vi "Step_Forward.vi"(3 "error in":errorcluster, 4 "Data in":T1, 5 "Step control reference in":refnum<vi>) -> (0 "error out":errorcluster, 1 "Data out":T1, 2 "Step control reference out":refnum<vi>)   [LabVIEW 2017]
uses:
  Type_Defs/Data.ctl
  Type_Defs/Diagnostics.ctl
  Type_Defs/Systems.ctl
  Step_Vis/Steps.lvlib
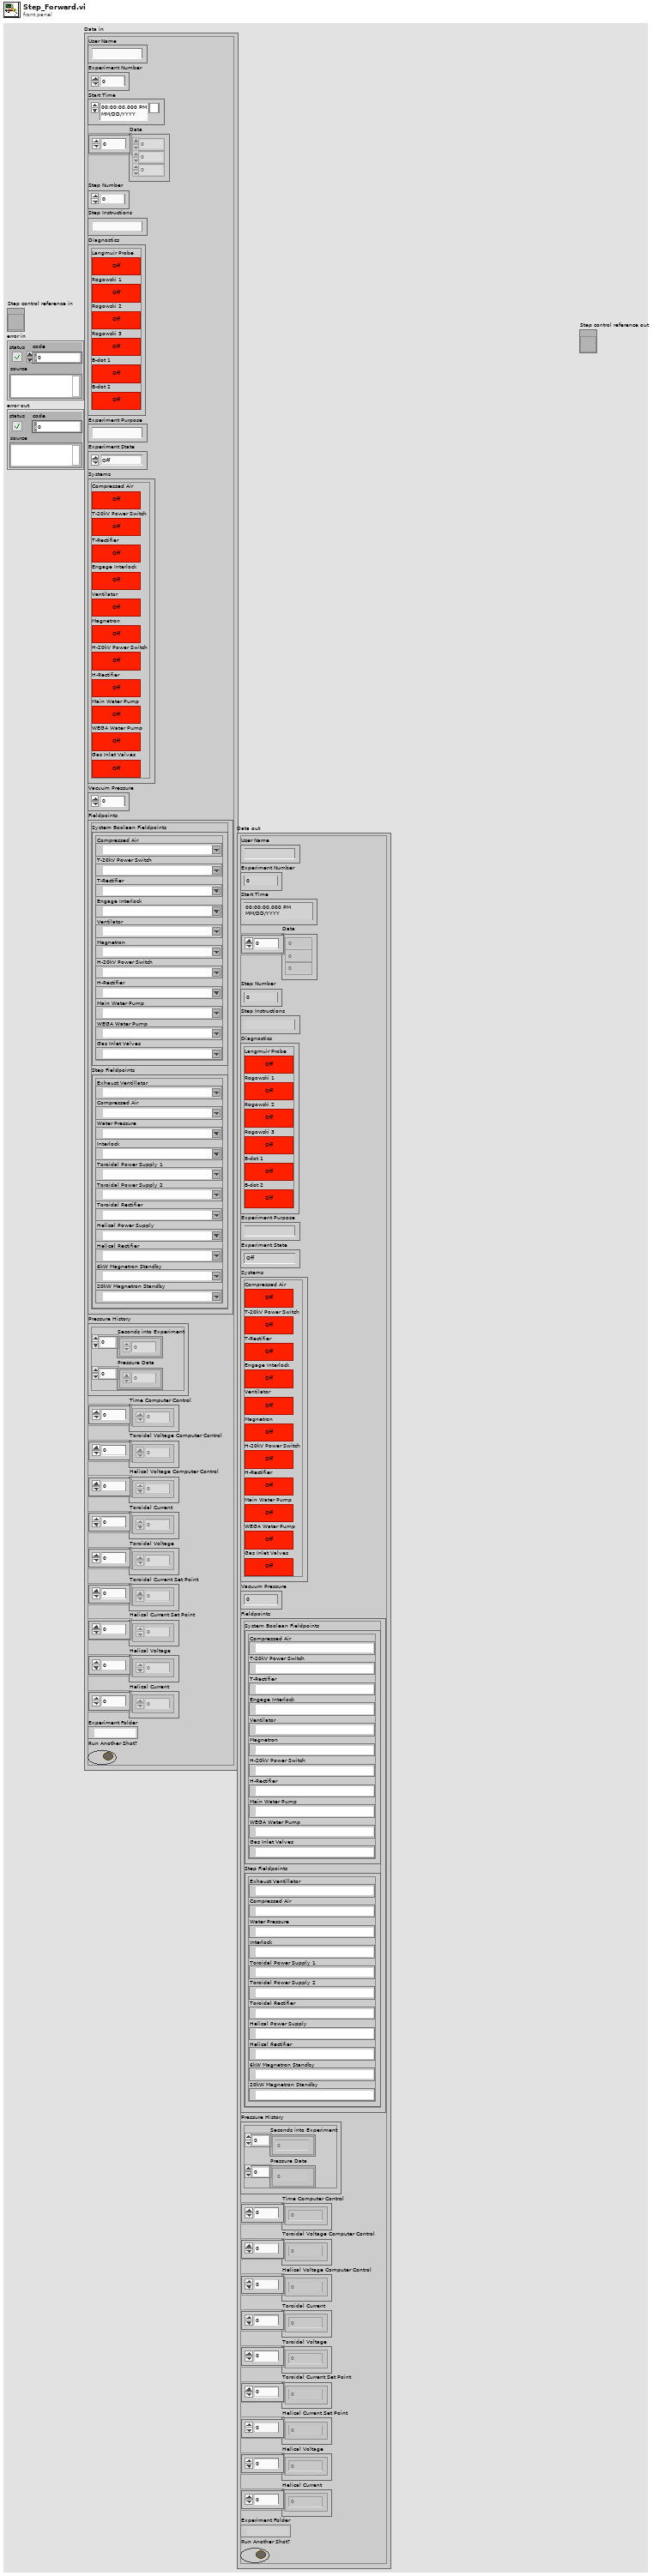
[diagram p1: front panel]
types:
  T1 = typedef "Data.ctl" = cluster{"User Name":string, "Experiment Number":i32, "Start Time":timestamp, "Data":dbl[], "Step Number":i32, "Step Instructions":string, "Diagnostics":T2, "Experiment Purpose":string, "Experiment State":enum16{"Off", "Setting Up", "Ready", "In Progress", "Shutting Down"}, "Systems":T3, "Vacuum Pressure":dbl, "Fieldpoints":cluster{"System Boolean Fieldpoints":cluster{"Compressed Air":refnum<k21>, "T-20kV Power Switch":refnum<k21>, "T-Rectifier":refnum<k21>, "Engage Interlock":refnum<k21>, "Ventilator":refnum<k21>, "Magnetron":refnum<k21>, "H-20kV Power Switch":refnum<k21>, "H-Rectifier":refnum<k21>, "Main Water Pump":refnum<k21>, "WEGA Water Pump":refnum<k21>, "Gas Inlet Valves":refnum<k21>}, "Step Fieldpoints":cluster{"Exhaust Ventillator":refnum<k21>, "Compressed Air":refnum<k21>, "Water Pressure":refnum<k21>, "Interlock":refnum<k21>, "Toroidal Power Supply 1":refnum<k21>, "Toroidal Power Supply 2":refnum<k21>, "Toroidal Rectifier":refnum<k21>, "Helical Power Supply":refnum<k21>, "Helical Rectifier":refnum<k21>, "6kW Magnetron Standby":refnum<k21>, "20kW Magnetron Standby":refnum<k21>}}, "Pressure History":cluster{"Seconds into Experiment":i32[], "Pressure Data":dbl[]}, "Time Computer Control":dbl[], "Toroidal Voltage Computer Control":dbl[], "Helical Voltage Computer Control":dbl[], "Toroidal Current":dbl[], "Toroidal Voltage":dbl[], "Toroidal Current Set Point":dbl[], "Helical Current Set Point":dbl[], "Helical Voltage":dbl[], "Helical Current":dbl[], "Experiment Folder":path, "Run Another Shot?":bool}
  T2 = typedef "Diagnostics.ctl" = cluster{"Langmuir Probe":bool, "Rogowski 1":bool, "Rogowski 2":bool, "Rogowski 3":bool, "B-dot 1":bool, "B-dot 2":bool}
  T3 = typedef "Systems.ctl" = cluster{"Compressed Air":bool, "T-20kV Power Switch":bool, "T-Rectifier":bool, "Engage Interlock":bool, "Ventilator":bool, "Magnetron":bool, "H-20kV Power Switch":bool, "H-Rectifier":bool, "Main Water Pump":bool, "WEGA Water Pump":bool, "Gas Inlet Valves":bool}
  T4 = enum16{"Off", "Setting Up", "Ready", "In Progress", "Shutting Down"}
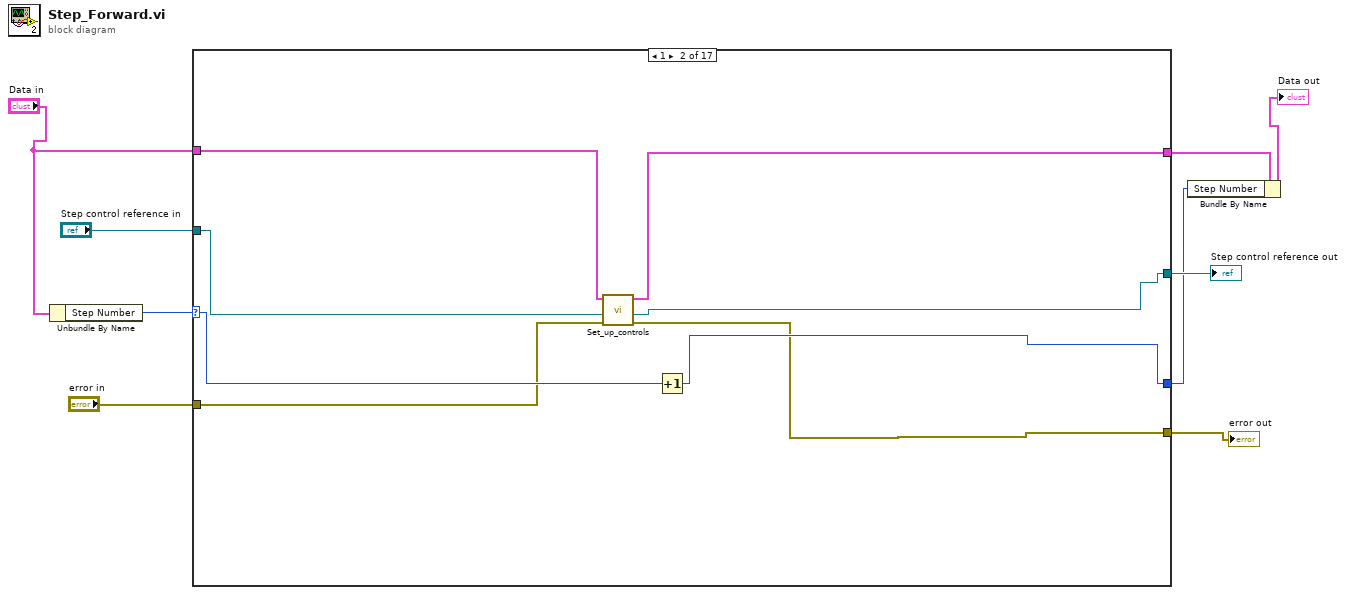
[diagram p0: block diagram]
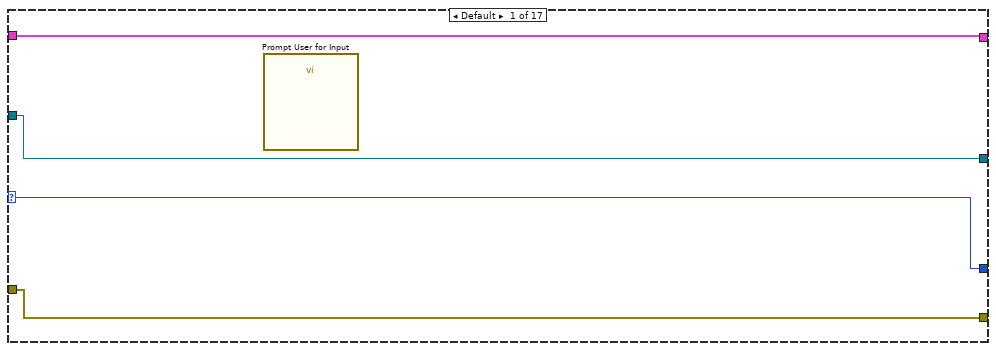
[diagram p2: hidden frame]
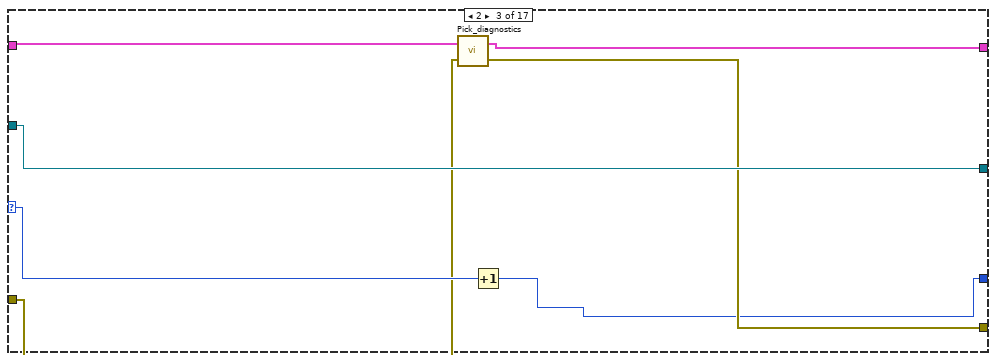
[diagram p3: hidden frame]
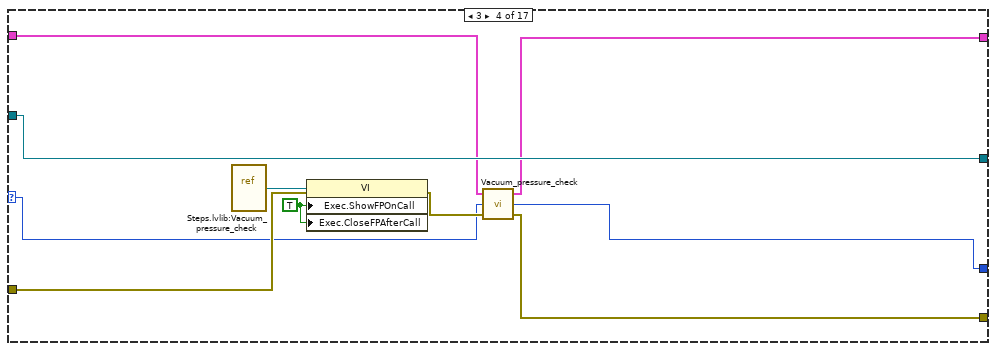
[diagram p4: hidden frame]
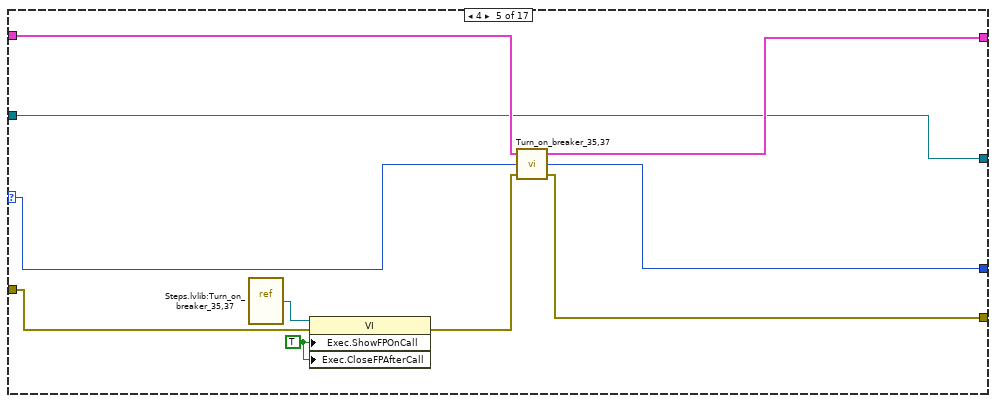
[diagram p5: hidden frame]
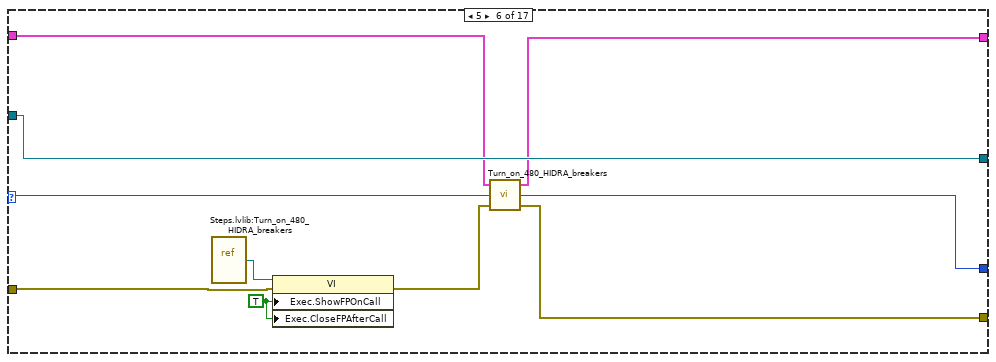
[diagram p6: hidden frame]
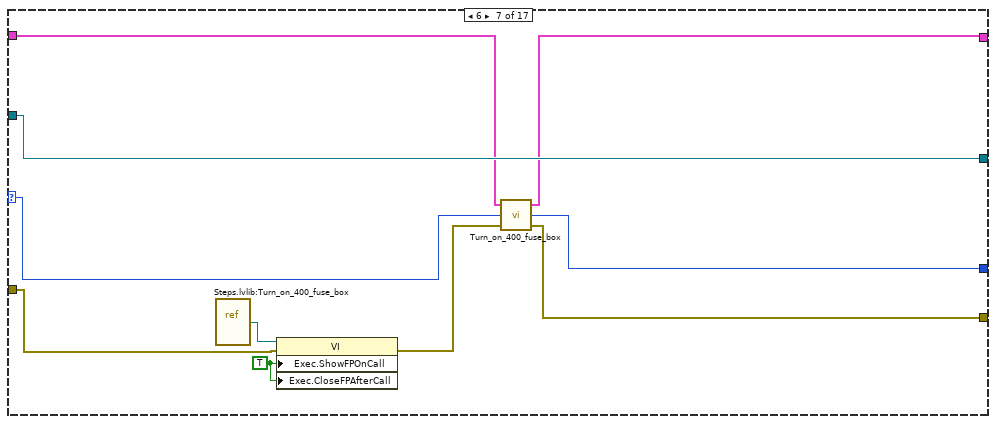
[diagram p7: hidden frame]
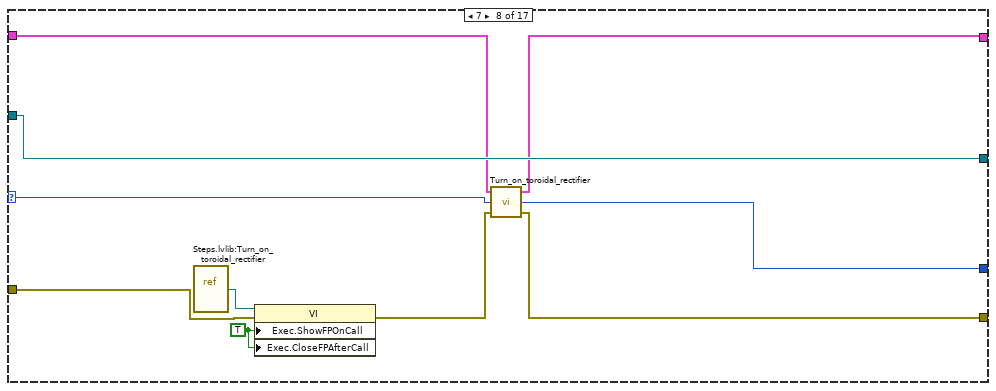
[diagram p8: hidden frame]
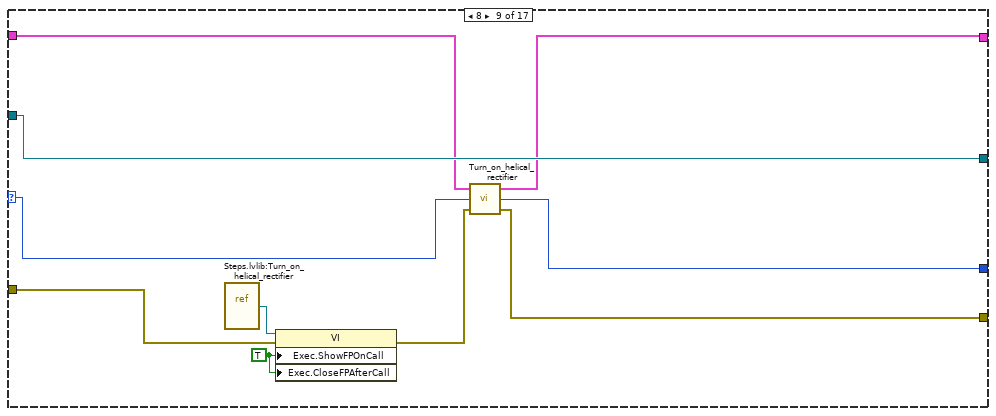
[diagram p9: hidden frame]
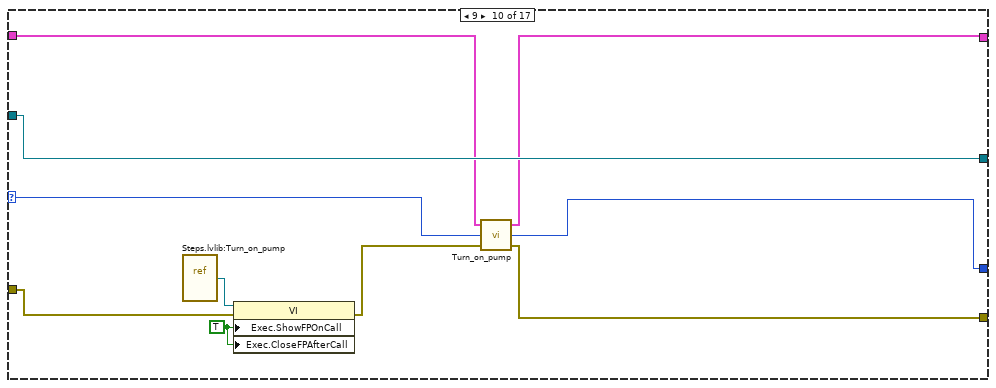
[diagram p10: hidden frame]
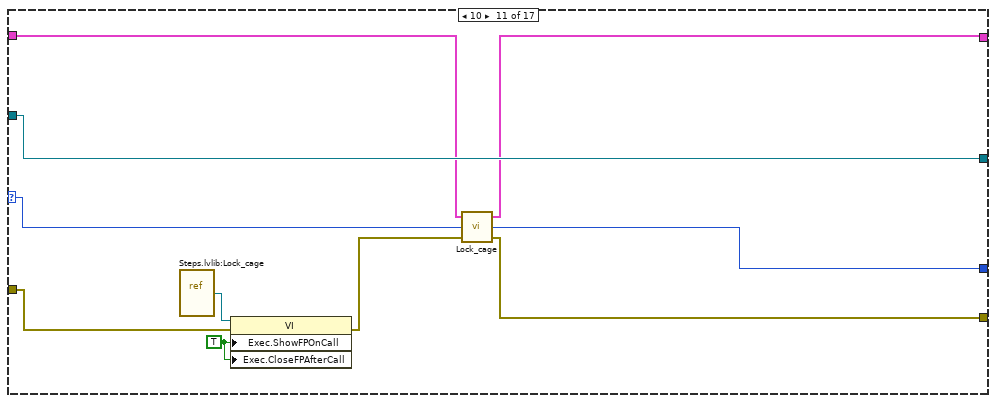
[diagram p11: hidden frame]
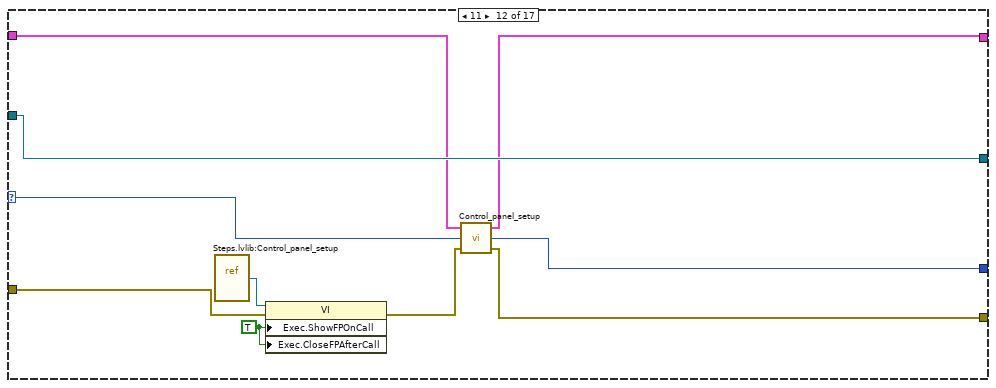
[diagram p12: hidden frame]
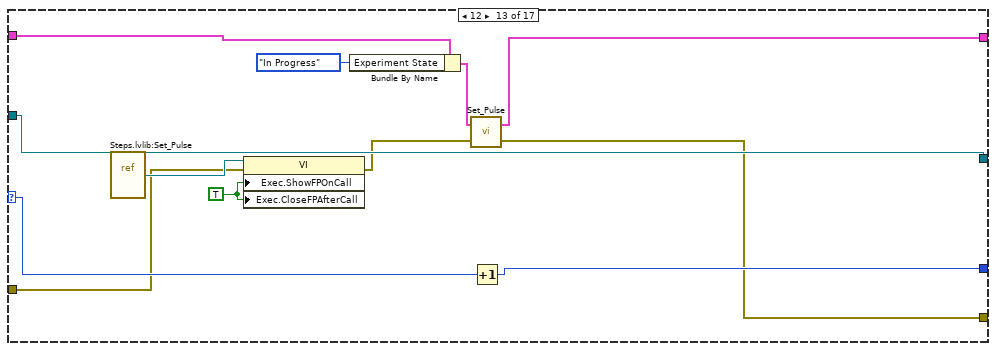
[diagram p13: hidden frame]
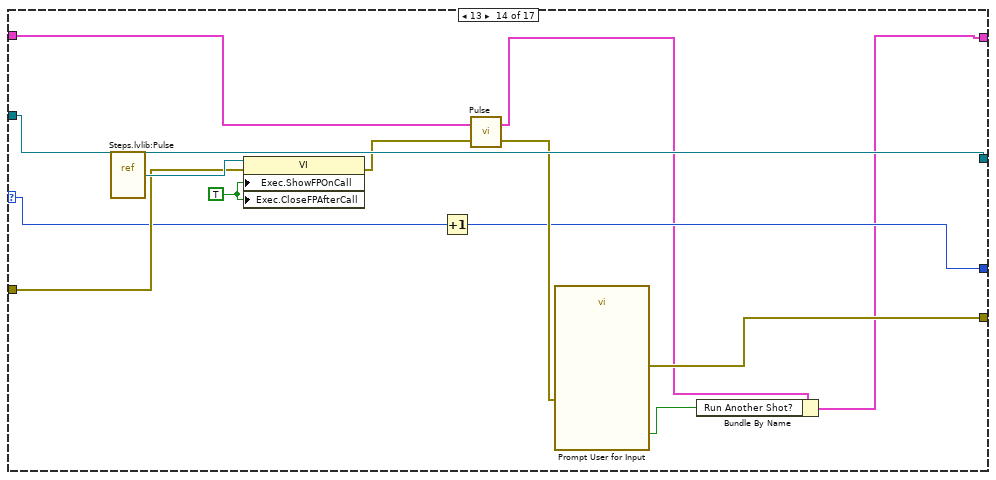
[diagram p14: hidden frame]
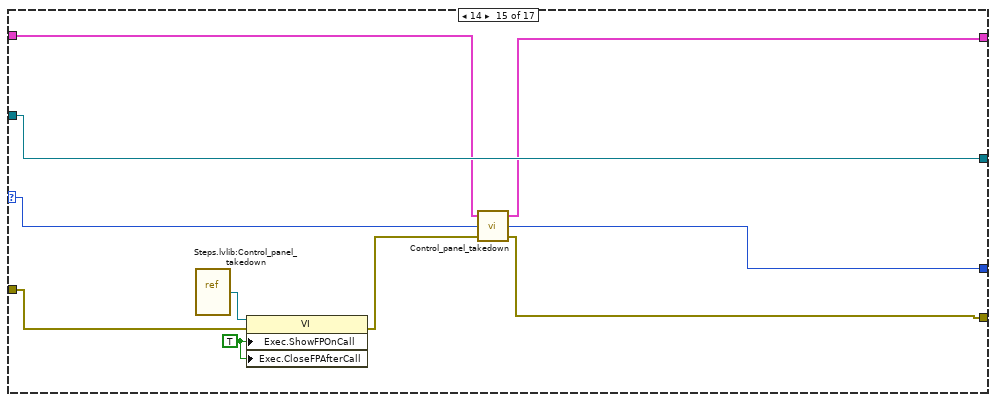
[diagram p15: hidden frame]
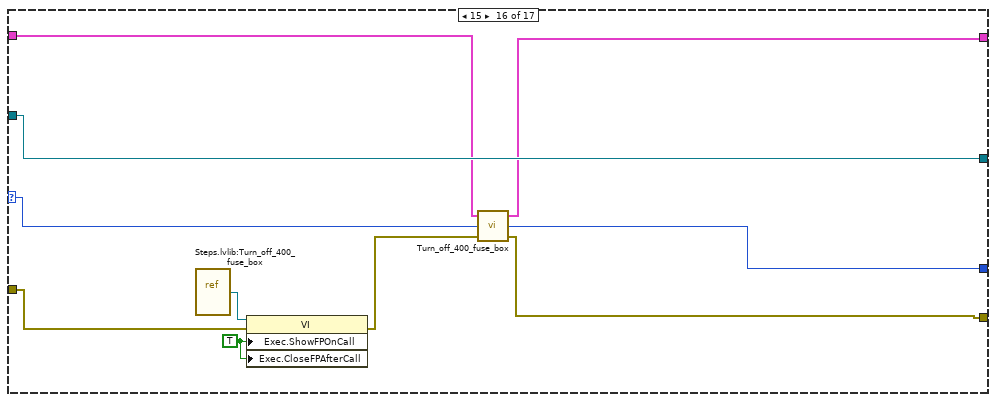
[diagram p16: hidden frame]
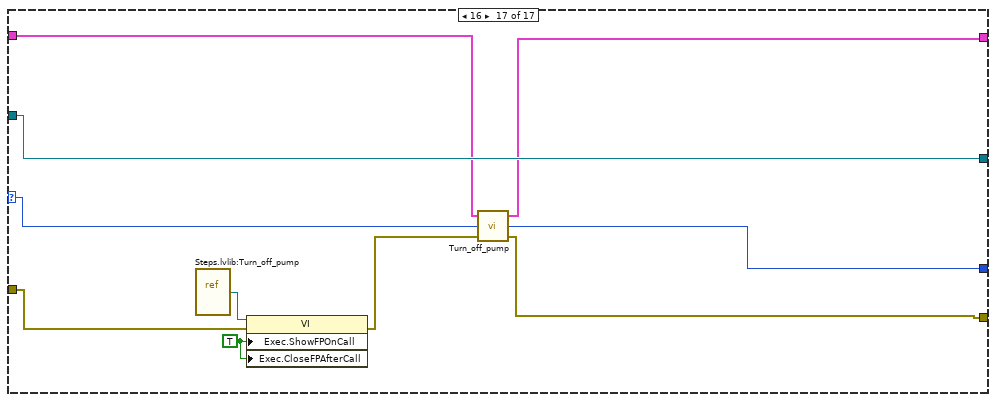
[diagram p17: hidden frame]
diagram:
  n1 = Unbundle By Name("Data in") -> ("Step Number"=w5:i32)
  n2 = case shown="1" w5 {
    selector: w5 -> [w12 w21 w28 w29 w45 w57 w65 w73 w85 w91 w102 w113 w128 w134 w146 w156 w166]
    tunnel: "Step control reference in" -> [w13 w19 w27 w38 w44 w58 w68 w78 w88 w98 w108 w118 w130 w143 w153 w163 w173]
    tunnel: [w13 w16 w27 w38 w44 w58 w68 w78 w88 w98 w108 w118 w130 w143 w153 w163 w173] -> w8
    tunnel: [w12 w15 w22 w30 w46 w53 w64 w74 w84 w92 w101 w112 w129 w135 w147 w157 w167] -> w3
    tunnel: "error in" -> [w11 w20 w23 w36 w41 w49 w59 w69 w82 w95 w105 w109 w124 w139 w149 w159 w169]
    tunnel: [w11 w14 w26 w34 w43 w54 w63 w75 w80 w93 w103 w111 w122 w136 w148 w158 w168] -> w6
    tunnel: "Data in" -> [w10 w18 w25 w32 w48 w55 w67 w77 w87 w90 w100 w115 w120 w140 w145 w155 w165]
    tunnel: [w10 w17 w24 w31 w47 w56 w66 w76 w86 w89 w99 w114 w125 w132 w144 w154 w164] -> w4
    frame Default {
      n3 = call "Prompt User for Input"() -> ()  [unwired: 18 in, 2 out]
    }
    frame 1 {
      n4 = call "Set_up_controls.vi"("error in"=w20, "reference"=w19, "Data in"=w18) -> ("error out"=w14:errorcluster, "reference out"=w16:refnum<vi>, "Data out"=w17:T1)  [unwired: 1 in, 1 out]
      n5 = Increment(x=w21) -> (x+1=w15:i32)
    }
    frame 2 {
      n6 = call "Pick_diagnostics.vi"("error in (no error)"=w23, "Data In"=w25) -> ("error out"=w26:errorcluster, "Data Out"=w24:T1)
      n7 = Increment(x=w28) -> (x+1=w22:i32)
    }
    frame 3 {
      w33 = TRUE ("Execution:Show Front Panel On Call")
      n8 = vi-ref "Steps.lvlib:Vacuum_pressure_check.vi"() -> (w37:refnum<vi>)
      n9 = property class="VI"(reference=w37, error in=w36, "Exec.ShowFPOnCall"=w33, "Exec.CloseFPAfterCall"=w33) -> (error out=w35:errorcluster)  [unwired: 1 out]
      n10 = call "Vacuum_pressure_check.vi"("error in"=w35, "Step Number in"=w29, "Data in"=w32) -> ("error out"=w34:errorcluster, "Step Number out"=w30:i32, "Data out"=w31:T1)
    }
    frame 4 {
      w42 = TRUE ("Execution:Show Front Panel On Call")
      n11 = vi-ref "Steps.lvlib:Turn_on_breaker_35,37.vi"() -> (w39:refnum<vi>)
      n12 = property class="VI"(reference=w39, error in=w41, "Exec.ShowFPOnCall"=w42, "Exec.CloseFPAfterCall"=w42) -> (error out=w40:errorcluster)  [unwired: 1 out]
      n13 = call "Turn_on_breaker_35,37.vi"("error in"=w40, "Step Number in"=w45, "Data in"=w48) -> ("error out"=w43:errorcluster, "Step Number out"=w46:i32, "Data out"=w47:T1)
    }
    frame 5 {
      w52 = TRUE ("Execution:Show Front Panel On Call")
      n14 = vi-ref "Steps.lvlib:Turn_on_480_HIDRA_breakers.vi"() -> (w51:refnum<vi>)
      n15 = property class="VI"(reference=w51, error in=w49, "Exec.ShowFPOnCall"=w52, "Exec.CloseFPAfterCall"=w52) -> (error out=w50:errorcluster)  [unwired: 1 out]
      n16 = call "Turn_on_480_HIDRA_breakers.vi"("error in"=w50, "Step Number in"=w57, "Data in"=w55) -> ("error out"=w54:errorcluster, "Step Number out"=w53:i32, "Data out"=w56:T1)
    }
    frame 6 {
      w62 = TRUE ("Execution:Show Front Panel On Call")
      n17 = vi-ref "Steps.lvlib:Turn_on_400_fuse_box.vi"() -> (w61:refnum<vi>)
      n18 = property class="VI"(reference=w61, error in=w59, "Exec.ShowFPOnCall"=w62, "Exec.CloseFPAfterCall"=w62) -> (error out=w60:errorcluster)  [unwired: 1 out]
      n19 = call "Turn_on_400_fuse_box.vi"("error in"=w60, "Step Number in"=w65, "Data in"=w67) -> ("error out"=w63:errorcluster, "Step Number out"=w64:i32, "Data out"=w66:T1)
    }
    frame 7 {
      w71 = TRUE ("Execution:Show Front Panel On Call")
      n20 = vi-ref "Steps.lvlib:Turn_on_toroidal_rectifier.vi"() -> (w72:refnum<vi>)
      n21 = property class="VI"(reference=w72, error in=w69, "Exec.ShowFPOnCall"=w71, "Exec.CloseFPAfterCall"=w71) -> (error out=w70:errorcluster)  [unwired: 1 out]
      n22 = call "Turn_on_toroidal_rectifier.vi"("error in"=w70, "Step Number in"=w73, "Data in"=w77) -> ("error out"=w75:errorcluster, "Step Number out"=w74:i32, "Data out"=w76:T1)
    }
    frame 8 {
      w83 = TRUE ("Execution:Show Front Panel On Call")
      n23 = vi-ref "Steps.lvlib:Turn_on_helical_rectifier.vi"() -> (w79:refnum<vi>)
      n24 = property class="VI"(reference=w79, error in=w82, "Exec.ShowFPOnCall"=w83, "Exec.CloseFPAfterCall"=w83) -> (error out=w81:errorcluster)  [unwired: 1 out]
      n25 = call "Turn_on_helical_rectifier.vi"("error in"=w81, "Step Number in"=w85, "Data in"=w87) -> ("error out"=w80:errorcluster, "Step Number out"=w84:i32, "Data out"=w86:T1)
    }
    frame 9 {
      w97 = TRUE ("Execution:Show Front Panel On Call")
      n26 = vi-ref "Steps.lvlib:Turn_on_pump.vi"() -> (w96:refnum<vi>)
      n27 = property class="VI"(reference=w96, error in=w95, "Exec.ShowFPOnCall"=w97, "Exec.CloseFPAfterCall"=w97) -> (error out=w94:errorcluster)  [unwired: 1 out]
      n28 = call "Turn_on_pump.vi"("error in"=w94, "Step Number in"=w91, "Data in"=w90) -> ("error out"=w93:errorcluster, "Step Number out"=w92:i32, "Data out"=w89:T1)
    }
    frame 10 {
      w106 = TRUE ("Execution:Show Front Panel On Call")
      n29 = vi-ref "Steps.lvlib:Lock_cage.vi"() -> (w107:refnum<vi>)
      n30 = property class="VI"(reference=w107, error in=w105, "Exec.ShowFPOnCall"=w106, "Exec.CloseFPAfterCall"=w106) -> (error out=w104:errorcluster)  [unwired: 1 out]
      n31 = call "Lock_cage.vi"("error in"=w104, "Step Number in"=w102, "Data in"=w100) -> ("error out"=w103:errorcluster, "Step Number out"=w101:i32, "Data out"=w99:T1)
    }
    frame 11 {
      w116 = TRUE ("Execution:Show Front Panel On Call")
      n32 = vi-ref "Steps.lvlib:Control_panel_setup.vi"() -> (w117:refnum<vi>)
      n33 = property class="VI"(reference=w117, error in=w109, "Exec.ShowFPOnCall"=w116, "Exec.CloseFPAfterCall"=w116) -> (error out=w110:errorcluster)  [unwired: 1 out]
      n34 = call "Control_panel_setup.vi"("error in"=w110, "Step Number in"=w113, "Data in"=w115) -> ("error out"=w111:errorcluster, "Step Number out"=w112:i32, "Data out"=w114:T1)
    }
    frame 12 {
      w127 = TRUE ("Execution:Show Front Panel On Call")
      n35 = vi-ref "Steps.lvlib:Set_Pulse.vi"() -> (w126:refnum<vi>)
      n36 = property class="VI"(reference=w126, error in=w124, "Exec.ShowFPOnCall"=w127, "Exec.CloseFPAfterCall"=w127) -> (error out=w123:errorcluster)  [unwired: 1 out]
      n37 = Bundle By Name(cluster=w120, "Experiment State"=T4."In Progress") -> (w119:T1)
      n38 = call "Set_Pulse.vi"("error in"=w123, "Data in"=w119) -> ("error out"=w122:errorcluster, "Data out"=w125:T1)
      n39 = Increment(x=w128) -> (x+1=w129:i32)
    }
    frame 13 {
      w142 = TRUE ("Execution:Show Front Panel On Call")
      n40 = vi-ref "Steps.lvlib:Pulse.vi"() -> (w141:refnum<vi>)
      n41 = property class="VI"(reference=w141, error in=w139, "Exec.ShowFPOnCall"=w142, "Exec.CloseFPAfterCall"=w142) -> (error out=w138:errorcluster)  [unwired: 1 out]
      n42 = Increment(x=w134) -> (x+1=w135:i32)
      n43 = call "Pulse.vi"("error in"=w138, "Data in"=w140) -> ("error out"=w137:errorcluster, "Data out"=w133:T1)
      n44 = call "Prompt User for Input"("error in (no error)"=w137) -> ("Run New Shot"=w131:bool, "error out"=w136:errorcluster)  [unwired: 16 in, 1 out]
      n45 = Bundle By Name(cluster=w133, "Run Another Shot?"=w131) -> (w132:T1)
    }
    frame 14 {
      w151 = TRUE ("Execution:Show Front Panel On Call")
      n46 = vi-ref "Steps.lvlib:Control_panel_takedown.vi"() -> (w152:refnum<vi>)
      n47 = property class="VI"(reference=w152, error in=w149, "Exec.ShowFPOnCall"=w151, "Exec.CloseFPAfterCall"=w151) -> (error out=w150:errorcluster)  [unwired: 1 out]
      n48 = call "Control_panel_takedown.vi"("error in"=w150, "Step Number in"=w146, "Data in"=w145) -> ("error out"=w148:errorcluster, "Step Number out"=w147:i32, "Data out"=w144:T1)
    }
    frame 15 {
      w161 = TRUE ("Execution:Show Front Panel On Call")
      n49 = vi-ref "Steps.lvlib:Turn_off_400_fuse_box.vi"() -> (w162:refnum<vi>)
      n50 = property class="VI"(reference=w162, error in=w159, "Exec.ShowFPOnCall"=w161, "Exec.CloseFPAfterCall"=w161) -> (error out=w160:errorcluster)  [unwired: 1 out]
      n51 = call "Turn_off_400_fuse_box.vi"("error in"=w160, "Step Number in"=w156, "Data in"=w155) -> ("error out"=w158:errorcluster, "Step Number out"=w157:i32, "Data out"=w154:T1)
    }
    frame 16 {
      w171 = TRUE ("Execution:Show Front Panel On Call")
      n52 = vi-ref "Steps.lvlib:Turn_off_pump.vi"() -> (w172:refnum<vi>)
      n53 = property class="VI"(reference=w172, error in=w169, "Exec.ShowFPOnCall"=w171, "Exec.CloseFPAfterCall"=w171) -> (error out=w170:errorcluster)  [unwired: 1 out]
      n54 = call "Turn_off_pump.vi"("error in"=w170, "Step Number in"=w166, "Data in"=w165) -> ("error out"=w168:errorcluster, "Step Number out"=w167:i32, "Data out"=w164:T1)
    }
  }
  "Step control reference out" <- w8
  "error out" <- w6
  n55 = Bundle By Name(cluster=w4, "Step Number"=w3) -> (→"Data out":T1)
